vi "GetAllAnalogInputVals.vi"(8 "error in (no error)":errorcluster, 11 "SerialPortRef":T1) -> (0 "error out":errorcluster, 1 "ADC raw values":u32[](array[numeric]) format="%012b", 2 "ADC voltages":dbl[](array[numeric]), 3 "SerialPortRef 2":T1)   [LabVIEW 2015]
uses:
  <vilib>/Rock Robotics/WPI/SerialPort/WPI_SerialPortRef.ctl
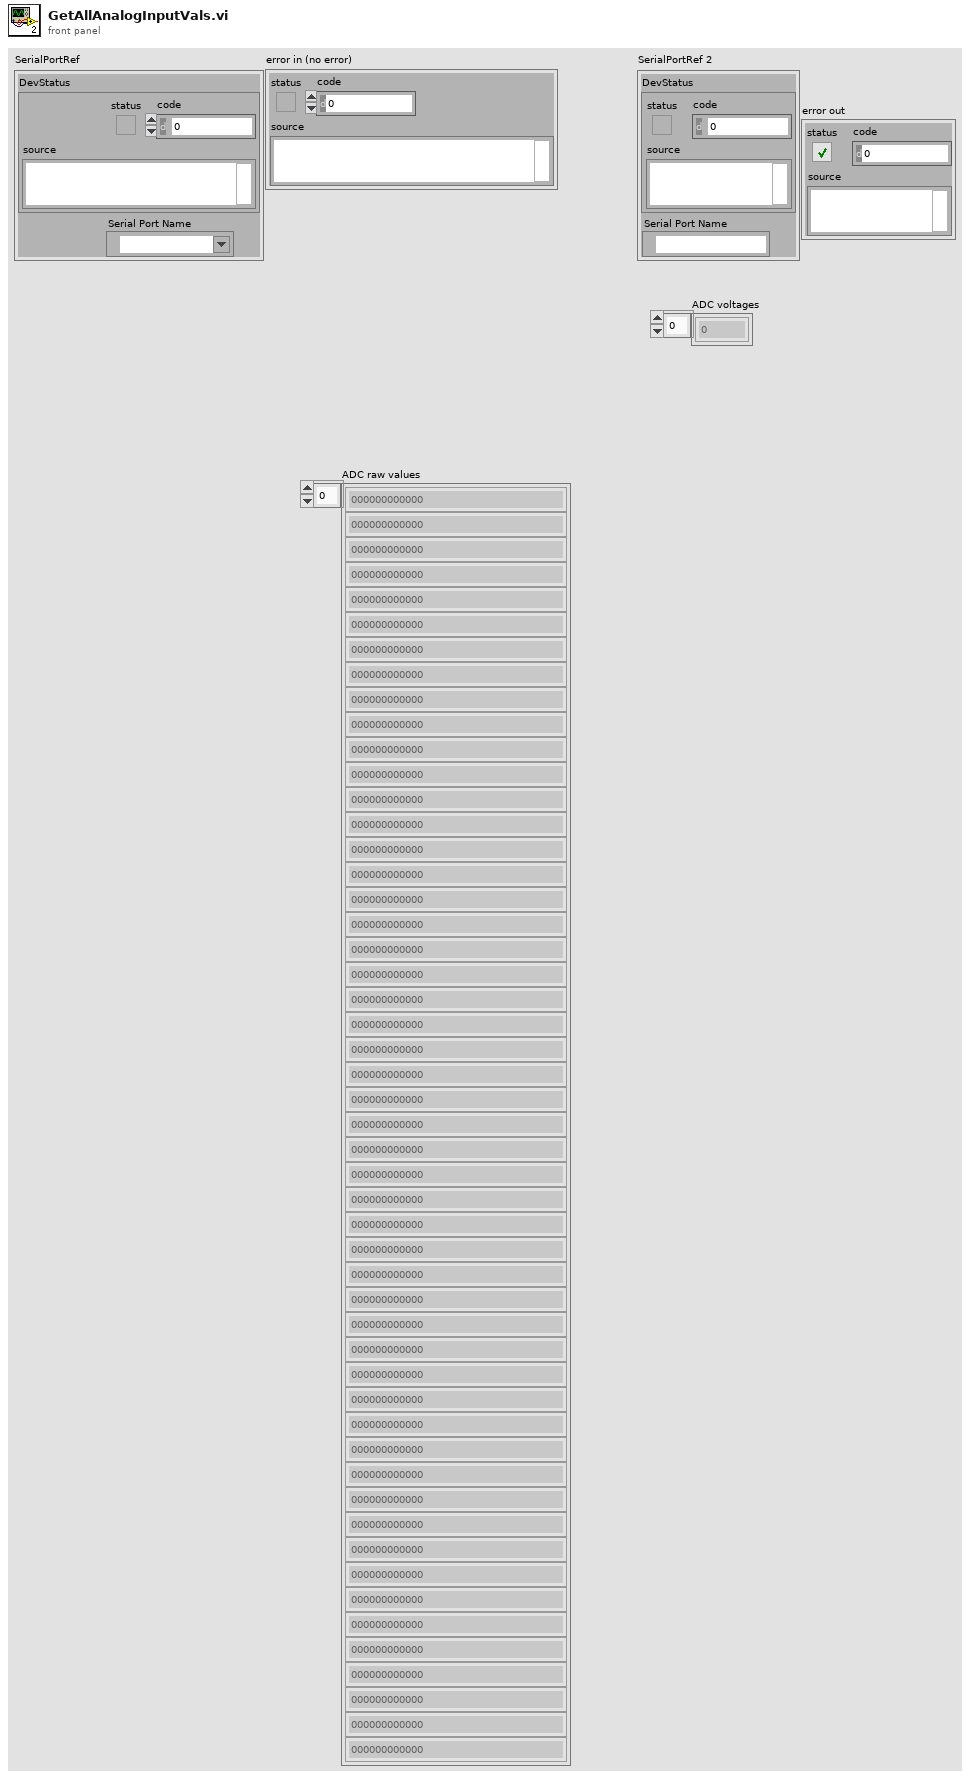
[diagram p1: front panel]
types:
  T1 = typedef "WPI_SerialPortRef.ctl" = cluster{"DevStatus":errorcluster, "Serial Port Name":refnum<visa-resource-name>}
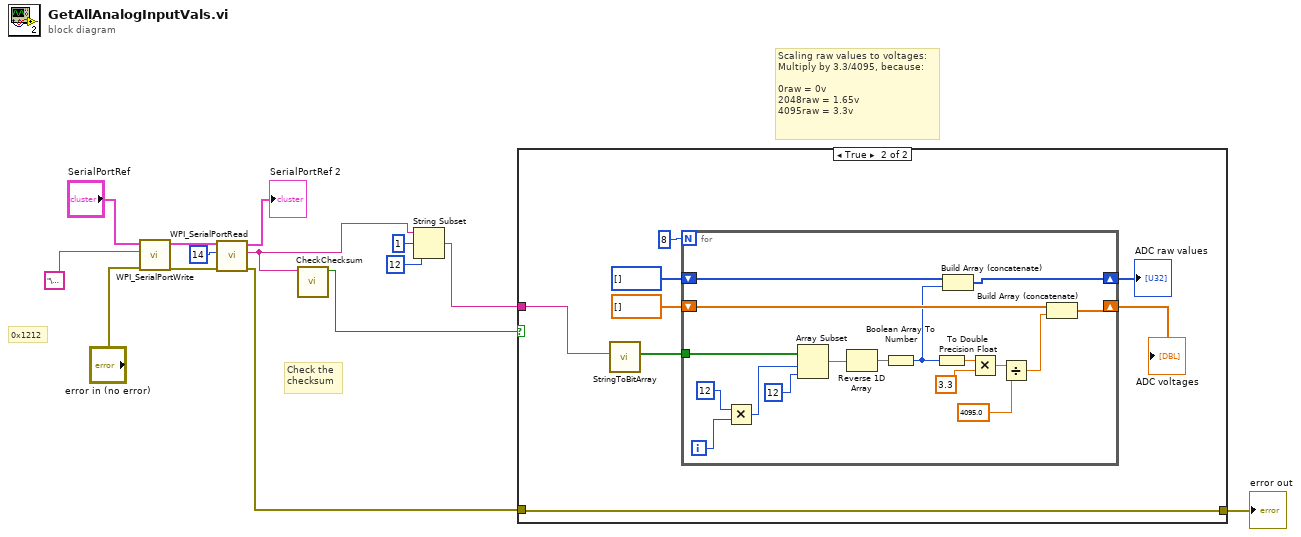
[diagram p0: block diagram]
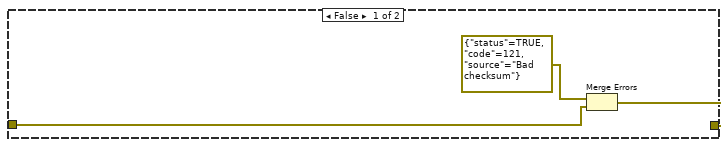
[diagram p2: hidden frame]
diagram:
  # "Scaling raw values to voltages:\nMultiply by 3.3/4095, because:\n\n0raw = 0v\n2048raw = 1.65v\n4095raw = 3.3v"
  # "Check the\nchecksum"
  # "0x1212"
  n1 = call <vilib>:"WPI_SerialPortWrite.vi"("error in (no error)"="error in (no error)", "Buffer"="\u0012", "SerialPortRef"="SerialPortRef") -> ("error out"=w5:errorcluster, "SerialPortRef"=w6:T1)  [unwired: 6 in, 1 out]
  n2 = call <vilib>:"WPI_SerialPortRead.vi"("error in (no error)"=w5, "Num Bytes to Read"=u32 14, "SerialPortRef"=w6) -> ("error out"=w1:errorcluster, "Buffer"=w3:string, "SerialPortRef"=→"SerialPortRef 2":T1)  [unwired: 6 in]
  n3 = call "CheckChecksum.vi"("String"=w3) -> ("x = y?"=w2:bool)  [unwired: 10 in]
  n4 = String Subset(string=w3, offset (0)=1, length (rest)=12 ("length (rest)")) -> (substring=w10:string)
  n5 = case shown="True" w2 {
    tunnel: w10 -> [_ w20]
    tunnel: w1 -> [w16 w25]
    tunnel: [w15 w25] -> w9
    frame False {
      n6 = Merge Errors(errorcluster {"status"=TRUE, "code"=121, "source"="Bad checksum"} ("error in"), w16) -> (w15:errorcluster)
    }
    frame True {
      n7 = call "StringToBitArray.vi"("string"=w20) -> ("Array"=w23:bool[])  [unwired: 10 in]
      n8 = for {
        N: 8 -> [_]
        tunnel: w23 -> [w42]
        shift-right: [w38] -> w21
        shift-left: u32[] [] -> [w37]
        shift-right: [w33] -> w18
        shift-left: dbl[] [] -> [w32]
        i -> [w41]
        n9 = Multiply(x=12, y=w41) -> (x*y=w39:i32)
        n10 = Array Subset(array=w42, index=w39, length=12) -> (w35:bool[])
        n11 = Reverse 1D Array(array=w35) -> (reversed array=w34:bool[])
        n12 = Boolean Array To Number(Boolean array=w34) -> (number=w26:u32)
        n13 = To Double Precision Float(number=w26) -> (double precision float=w27:dbl)
        n14 = Build Array (concatenate)(w37, w26) -> (w38:u32[])
        n15 = Multiply(x=w27, y=3.3) -> (x*y=w30:dbl)
        n16 = Divide(x=w30, y=4095.0) -> (x/y=w28:dbl)
        n17 = Build Array (concatenate)(w32, w28) -> (w33:dbl[])
      }
      "ADC raw values" <- w21
      "ADC voltages" <- w18
    }
  }
  "error out" <- w9
